vi "Find CRT Coincs.vi"(11 "Coincidences":T1[](array[typedef])) -> (0 "Good tracks":T2(array[cluster]), 2 "Single hits":T1[](array[typedef]), 3 "CRT-wide coincidences":cluster{"CRT-wide coincs":T1[]}[](array[cluster]))   [LabVIEW 2016]
uses:
  Typedefs/Coincidence.ctl
  Global Variables/Global Resolution.vi
  Global Variables/Coincidence Windows.vi
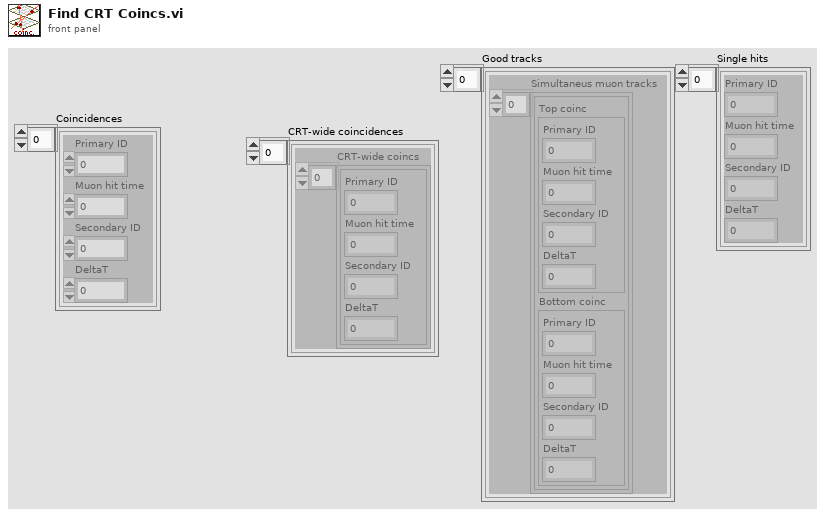
[diagram p1: front panel]
types:
  T1 = typedef "Coincidence.ctl" = cluster{"Primary ID":i8, "Muon hit time":u64, "Secondary ID":i8, "DeltaT":i32}
  T2 = cluster{"Simultaneus muon tracks":cluster{"Top coinc":T1, "Bottom coinc":T1}[]}[]
  T3 = cluster{"Primary ID":bool, "Muon hit time":bool, "Secondary ID":bool, "DeltaT":bool}
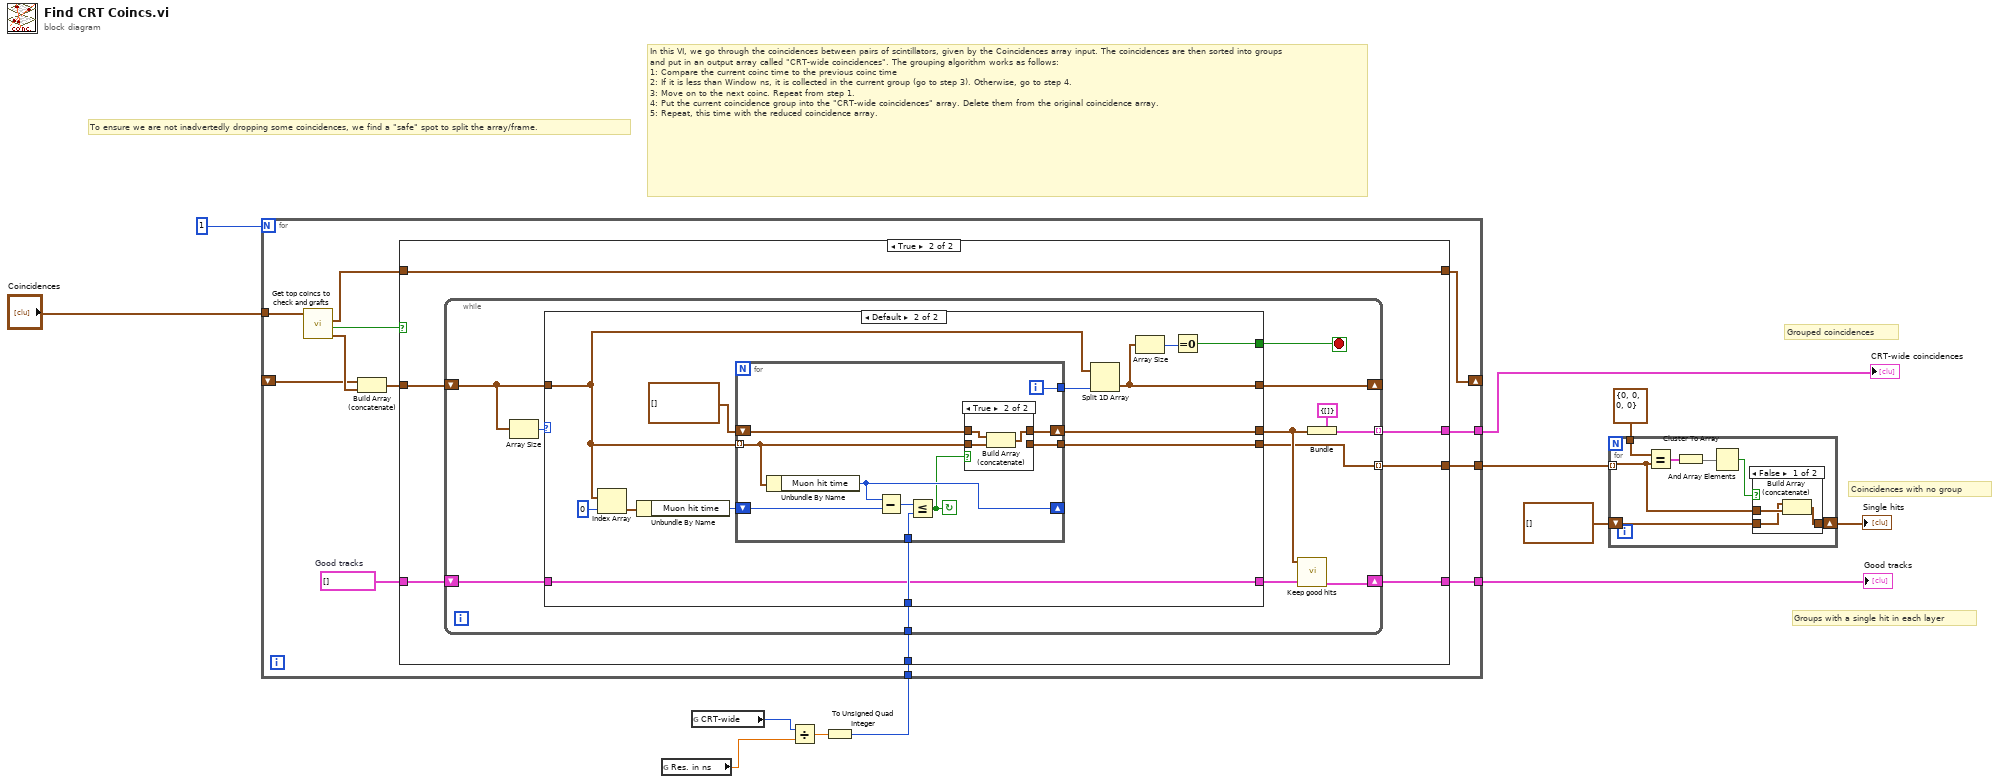
[diagram p0: block diagram]
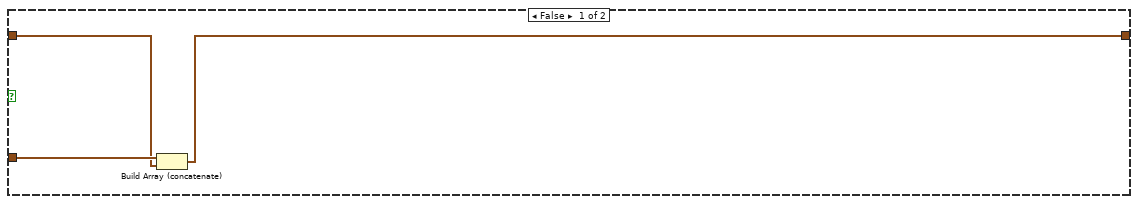
[diagram p3: hidden frame]
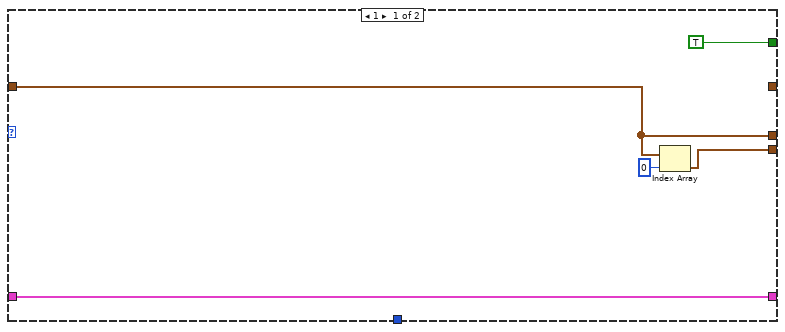
[diagram p4: hidden frame]
diagram:
  # "Groups with a single hit in each layer"
  # "Coincidences with no group"
  # "Grouped coincidences"
  # "To ensure we are not inadvertedly dropping some coincidences, we find a \"safe\" spot to split the array/frame."
  # "In this VI, we go through the coincidences between pairs of scintillators, given by the Coincidences array input. The coincidences are then sorted into groups and put in an output array called \"CRT-wide coincidences\". The grouping algorithm works as follows: \n1: Compare the current coinc time to the previous coinc time\n2: If it is less than Window ns, it is collected in the current group (go to step 3). Otherwise, go to step 4.\n3: Move on to the next coinc. Repeat from step 1.\n4: Put the current coincidence group into the \"CRT-wide coincidences\" array. Delete them from the original coincidence array.\n5: Repeat, this time with the reduced coincidence array."
  n1 = global read "Global Resolution.vi" "Res. in ns"() -> (w8:ext)
  n2 = global read "Coincidence Windows.vi" "CRT-wide"() -> (w1:i32)
  n3 = Divide(x=w1, y=w8) -> (x/y=w9:ext)
  n4 = To Unsigned Quad Integer(1:w9) -> (0:w11:u64)
  n5 = for {
    N: 1 -> [_]
    tunnel: "Coincidences" -> [w24]
    tunnel: w11 -> [w21]
    tunnel: [w20] -> w10
    tunnel: [w19] -> w6
    shift-right: [w15] -> _
    shift-left: _ -> [w18]
    tunnel: [w13] -> w5
    w17 = T2 []  # Good tracks
    n6 = call "Get top coincs to check and grafts.vi"("Coincidences"=w24) -> ("Coincidences to check"=w23:T1[], "Found safe graft spot?"=w16:bool, "Coincidences to graft"=w14:T1[])  [unwired: 8 in]
    n7 = Build Array (concatenate)(w18, w23) -> (w22:T1[])
    n8 = case shown="True" w16 {
      tunnel: w22 -> [w27 w34]
      tunnel: w21 -> [_ w33]
      tunnel: [_ w32] -> w20
      tunnel: [_ w31] -> w19
      tunnel: w17 -> [_ w30]
      tunnel: [w25 w29] -> w15
      tunnel: w14 -> [w26 w29]
      tunnel: [_ w28] -> w13
      frame False {
        n9 = Build Array (concatenate)(w27, w26) -> (w25:T1[])
      }
      frame True {
        n10 = while {
          tunnel: w33 -> [w46]
          shift-right: [w43] -> _
          shift-left: w34 -> [w40]
          tunnel: [w44] -> w32 mode=indexing
          shift-right: [w36] -> w31
          shift-left: w30 -> [w39]
          tunnel: [w35] -> w28 mode=indexing
          stop <- w42 stop-if-true
          n11 = Array Size(array=w40) -> (size(s)=w41:i32)
          n12 = case shown="Default" w41 {
            tunnel: w46 -> [_ w64]
            tunnel: [w49 w54] -> w37
            tunnel: w40 -> [w49 w60]
            tunnel: [_ w57] -> w43
            tunnel: [TRUE w55] -> w42
            tunnel: w39 -> [w50 w53]
            tunnel: [w50 w53] -> w38
            tunnel: [w47 w52] -> w35
            frame 1 {
              n13 = Index Array(array=w49, index=0) -> (element=w47:T1)
            }
            frame Default {
              n14 = Index Array(array=w60, index=0) -> (element=w59:T1)
              n15 = Unbundle By Name(w59) -> ("Muon hit time"=w61:u64)
              n16 = for {
                tunnel: w60 -> [w69] mode=indexing
                shift-right: [w74] -> _
                shift-left: w61 -> [w73]
                tunnel: w64 -> [w71]
                tunnel: [w66] -> w63
                shift-right: [w68] -> w54
                shift-left: T1[] [] -> [w67]
                tunnel: [w65] -> w52
                i -> [w66]
                stop <- w70 continue-if-true
                n17 = Unbundle By Name(w69) -> ("Muon hit time"=w74:u64)
                n18 = Subtract(x=w74, y=w73) -> (x-y=w72:u64)
                n19 = Less Or Equal?(x=w72, y=w71) -> (x <= y?=w70:bool)
                n20 = case shown="True" w70 {
                  tunnel: w69 -> [w75 w79]
                  tunnel: [w76 w78] -> w68
                  tunnel: w67 -> [w76 w77]
                  tunnel: [w75 _] -> w65
                  frame False {
                  }
                  frame True {
                    n21 = Build Array (concatenate)(w77, w79) -> (w78:T1[])
                  }
                }
              }
              n22 = Split 1D Array(array=w60, index=w63) -> (second subarray=w57:T1[])  [unwired: 1 out]
              n23 = Array Size(array=w57) -> (size(s)=w56:i32)
              n24 = Equal To 0?(x=w56) -> (x = 0?=w55:bool)
            }
          }
          n25 = call "Keep good hits.vi"("Collection in"=w38, "Array"=w37) -> ("Collection out"=w36:T2)  [unwired: 9 in]
          n26 = Bundle(cluster=cluster{"CRT-wide coincs":T1[]} {"CRT-wide coincs"=[]}, "CRT-wide coincs"=w37) -> (w44:cluster{"CRT-wide coincs":T1[]})
        }
      }
    }
  }
  "CRT-wide coincidences" <- w10
  "Good tracks" <- w6
  n27 = for {
    tunnel: w5 -> [w83] mode=indexing
    shift-right: [w81] -> w3
    shift-left: T1[] [] -> [w82]
    tunnel: T1 {"Primary ID"=0, "Muon hit time"=0, "Secondary ID"=0, "DeltaT"=0} ("Coincidence") -> [w80]
    n28 = Equal?(x=w80, y=w83) -> (x = y?=w86:T3)
    n29 = Cluster To Array(cluster=w86) -> (array=w85:bool[])
    n30 = And Array Elements(Boolean array=w85) -> (logical AND=w84:bool)
    n31 = case shown="False" w84 {
      tunnel: w83 -> [w89 _]
      tunnel: w82 -> [w88 w90]
      tunnel: [w87 w90] -> w81
      frame False {
        n32 = Build Array (concatenate)(w88, w89) -> (w87:T1[])
      }
      frame True {
      }
    }
  }
  "Single hits" <- w3
